vi "Get Channel Data.vi"(8 "error in (no error)":errorcluster, 9 "interface":refnum<k21>, 10 "signal list":refnum<k21>[](array[refnum]), 11 "PXI 8513 in":refnum<class "PXI 8513.lvclass">) -> (0 "error out":errorcluster, 2 "Data":dbl[](array[numeric]), 3 "PXI 8513 out":refnum<class "PXI 8513.lvclass">)   [LabVIEW 2016, in "CAN.lvlib" / "PXI 8513.lvclass"]
uses:
  PXI 8513.lvclass
  <vilib>/xnet/xnet.llb/XNET Create Session (Signal Input Single-point).vi
  <vilib>/xnet/xnet.llb/XNET Read (Signal Single-point).vi
  <resource>/objmgr/xnet.rc
  User Interface/User Interface.lvlib
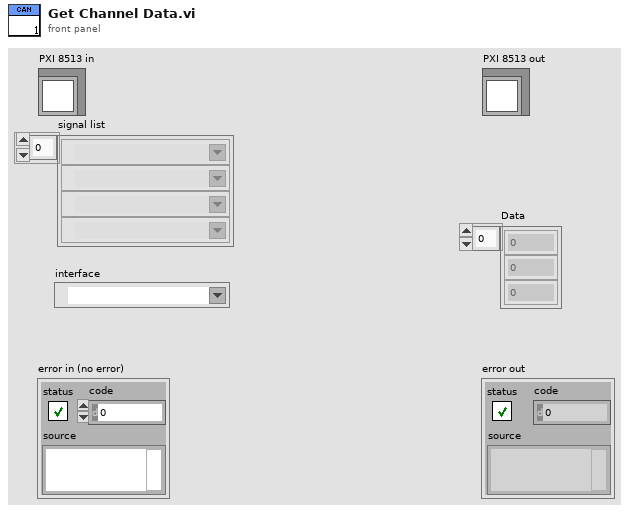
[diagram p1: front panel]
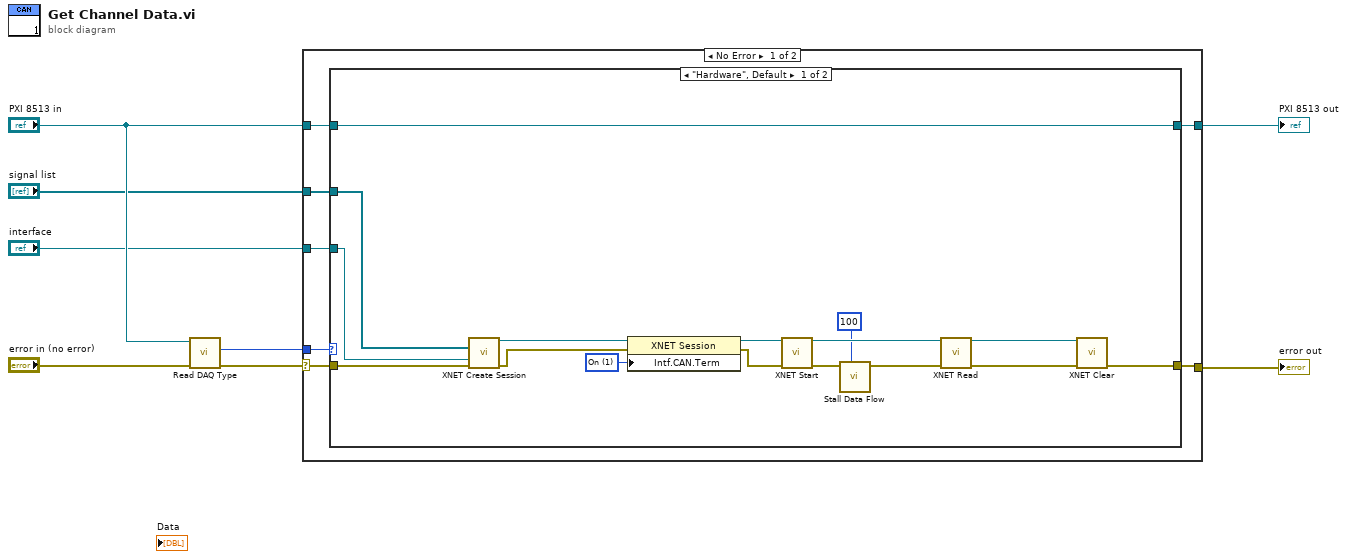
[diagram p0: block diagram]
diagram:
  n1 = call-dynamic "Read DAQ Type.vi"("error in (no error)"="error in (no error)", "PXI 8513 in"="PXI 8513 in") -> ("error out"=w7:errorcluster, "DAQ Type"=w6:enum16{"Hardware", "Simulation"})  [unwired: 7 in, 1 out]
  n2 = case shown="No Error" w7 {
    selector: w7 -> [w15 w34]
    tunnel: "PXI 8513 in" -> [w13 w35]
    tunnel: w6 -> [w14 _]
    tunnel: "signal list" -> [w12 _]
    tunnel: "interface" -> [w11 _]
    tunnel: [w10 w34] -> w2
    tunnel: [w9 w35] -> w1
    frame No Error {
      n3 = case shown="\"Hardware\", Default" w14 {
        tunnel: w15 -> [w31 w32]
        tunnel: w13 -> [w16 w33]
        tunnel: w12 -> [w30 _]
        tunnel: w11 -> [w29 _]
        tunnel: [w17 w32] -> w10
        tunnel: [w16 w33] -> w9
        frame "Hardware", Default {
          w27 = u32 1 items=["Off", "On"] ("Interface:CAN:Termination")
          n4 = call-poly <vilib>:"XNET Create Session.vi"("signal list"=w30, "interface"=w29, "error in (no error)"=w31) -> ("session out"=w28:refnum<k21>, "error out"=w26:errorcluster)  [unwired: 11 in]
          n5 = property class="XNET Session"(reference=w28, error in=w26, "Intf.CAN.Term"=w27) -> (reference out=w25:refnum<k21>, error out=w24:errorcluster)
          n6 = call <vilib>:"XNET Start.vi"("session in"=w25, "error in (no error)"=w24) -> ("session out"=w23:refnum<k21>, "error out"=w22:errorcluster)  [unwired: 12 in]
          n7 = call "Stall Data Flow.vi"("milliseconds to wait"=u32 100, "error in (no error)"=w22) -> ("error out"=w21:errorcluster)  [unwired: 9 in]
          n8 = call-poly <vilib>:"XNET Read.vi"("session in"=w23, "error in (no error)"=w21) -> ("session out"=w18:refnum<k21>, "error out"=w19:errorcluster)  [unwired: 11 in, 1 out]
          n9 = call <vilib>:"XNET Clear.vi"("session in"=w18, "error in (no error)"=w19) -> ("error out"=w17:errorcluster)  [unwired: 13 in]
        }
        frame "Simulation" {
        }
      }
    }
    frame Error {
    }
  }
  "error out" <- w2
  "PXI 8513 out" <- w1
